vi "Thermal Chamber Controller_DQMH_Action Update Set Point-teardown-Caraya.vi"(8 "error out":errorcluster, 11 "test case ID":string) -> (3 "result":bool)   [LabVIEW 2018]
doc: "The teardown VI should be executed after the VI under test in the harness VI. In this VI you can evaluate the outputs of the VI under test.\n\nSee the Help Document for more information. (<b>Help</b> > <b>IncQuery Labs</b> > <b>InstaCoverage</b> > <b>InstaCoverage Help...</b>)"
uses:
  Libraries/Thermal Chamber Response Simulator/Thermal Chamber Response Simulator.lvlib
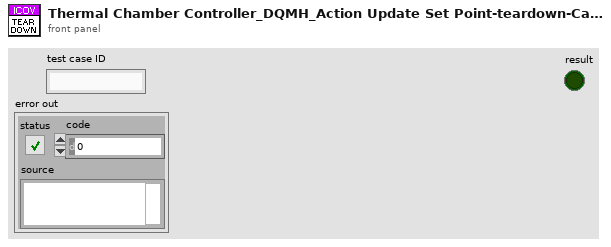
[diagram p1: front panel]
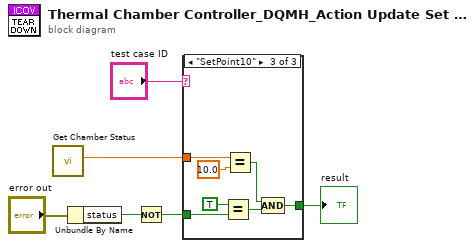
[diagram p0: block diagram]
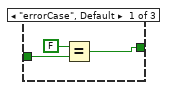
[diagram p2: hidden frame]
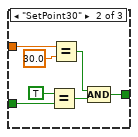
[diagram p3: hidden frame]
diagram:
  n1 = call "Get Chamber Status.vi"() -> ("Temperature Set Point (deg C)"=w3:dbl)  [unwired: 6 in, 5 out]
  n2 = Unbundle By Name("error out") -> ("status"=w6:bool)
  n3 = Not(x=w6) -> (.not. x?=w4:bool)
  n4 = case shown="\"SetPoint10\"" "test case ID" {
    tunnel: w4 -> [w7 w11 w23]
    tunnel: w3 -> [_ w12 w20]
    tunnel: [w8 w10 w17] -> w2
    frame "errorCase", Default {
      n5 = Equal?(x=FALSE, y=w7) -> (x = y?=w8:bool)
    }
    frame "SetPoint30" {
      n6 = Equal?(x=TRUE, y=w11) -> (x = y?=w13:bool)
      n7 = Equal?(x=w12, y=30.0) -> (x = y?=w14:bool)
      n8 = Compound Arithmetic op=AND(w14, w13) -> (w10:bool)
    }
    frame "SetPoint10" {
      n9 = Equal?(x=TRUE, y=w23) -> (x = y?=w18:bool)
      n10 = Equal?(x=w20, y=10.0) -> (x = y?=w19:bool)
      n11 = Compound Arithmetic op=AND(w19, w18) -> (w17:bool)
    }
  }
  "result" <- w2
